vi "Send Command.vi"(7 "VolatusAPI":refnum<class "VolatusAPI.lvclass">, 8 "error in (no error)":errorcluster, 10 "Value":dbl, 11 "DblPopupControl in":refnum<class "DblPopupControl.lvclass">) -> (0 "error out":errorcluster, 3 "DblPopupControl out":refnum<class "DblPopupControl.lvclass">)   [LabVIEW 2020, in "VolatusGUIElements.lvlib" / "DblPopupControl.lvclass"]
uses:
  DblPopupControl.lvclass
  Volatus/VolatusAPI/VolatusAPI.lvclass
  Cmd State.ctl
  DblPopupControl.lvclass/DblPopupControl.ctl
  messages/CmdAnalog/Class/Msg.lvclass/Msg.ctl
  Volatus/VolatusAPI/VolatusAPI.lvclass/VolatusAPI.ctl
  messages/CmdAnalog/Class/Msg.lvclass
  C:/dev/lv20CE/relink/lv-protoc/LV-Proto/Message/Message.lvclass
  lv-vecto/Vecto/TCPMessageService/Send Message.vi
  <vilib>/Utility/error.llb/Error Cluster From Error Code.vi
  lv-protoc/LV-Proto/Message/Message.lvclass
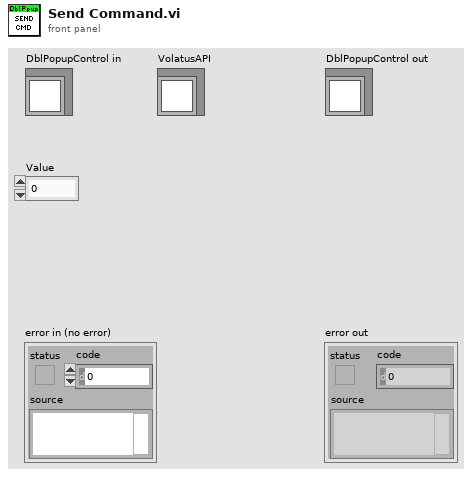
[diagram p1: front panel]
types:
  T1 = typedef "VolatusGUIElements.lvlib/DblPopupControl.lvclass/Cmd State.ctl" = cluster{"Commanding":bool, "Start":dbl, "Error":bool, "Value":dbl}
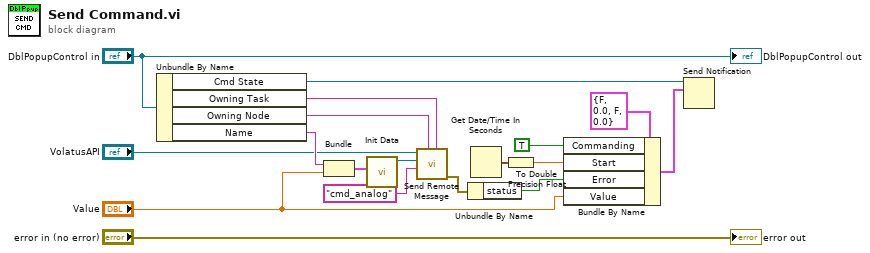
[diagram p0: block diagram]
diagram:
  n1 = Unbundle By Name("DblPopupControl in") -> ("Cmd State"=w9:refnum<notifier>, "Owning Task"=w10:string, "Owning Node"=w17:string, "Name"=w16:string)
  n2 = Bundle("Name"=w16, "Value"="Value") -> (w15:cluster{"Name":string, "Value":dbl})  [unwired: 1 in]
  n3 = call "Init Data.vi"("Data"=w15) -> ("Msg out"=w14:refnum<class "Msg.lvclass">)  [unwired: 10 in]
  n4 = call "Send Remote Message.vi"("Target Task (None)"=w10, "Target Node"=w17, "Message Type"="cmd_analog", "Message"=w14, "VolatusAPI in"="VolatusAPI") -> ("error out"=w3:errorcluster)  [unwired: 5 in, 1 out]
  n5 = Unbundle By Name(w3) -> ("status"=w2:bool)
  n6 = Get Date/Time In Seconds() -> (seconds since 1Jan1904=w6:timestamp)
  n7 = To Double Precision Float(number=w6) -> (double precision float=w5:dbl)
  n8 = Bundle By Name(cluster=T1 {"Commanding"=FALSE, "Start"=0.0, "Error"=FALSE, "Value"=0.0} ("notification"), "Commanding"=TRUE, "Start"=w5, "Error"=w2, "Value"="Value") -> (w7:T1)
  n9 = Send Notification(notification=w7, notifier=w9) -> ()  [unwired: 1 in, 2 out]
  "error out" <- "error in (no error)"
  "DblPopupControl out" <- "DblPopupControl in"
